vi "CMN_Algors.vi"(0 "ValueIn":string, 1 "file":path, 2 "algors":string[](array[string]), 3 "error in (no error)":errorcluster, 5 "action":T2(ring)) -> (7 "Value out":sgl format="%.6f", 9 "string value":string, 10 "error out":errorcluster)   [LabVIEW 2016]
uses:
  <vilib>/Utility/config.llb/Read Key (String).vi
  <vilib>/Utility/config.llb/NI_LVConfig.lvlib
panel:
  in  "algor":T1
  # "Hacer un <Window/SHOW DIAGRAM> para ver \nalgoritmos definidos o agregar uno nuevo"
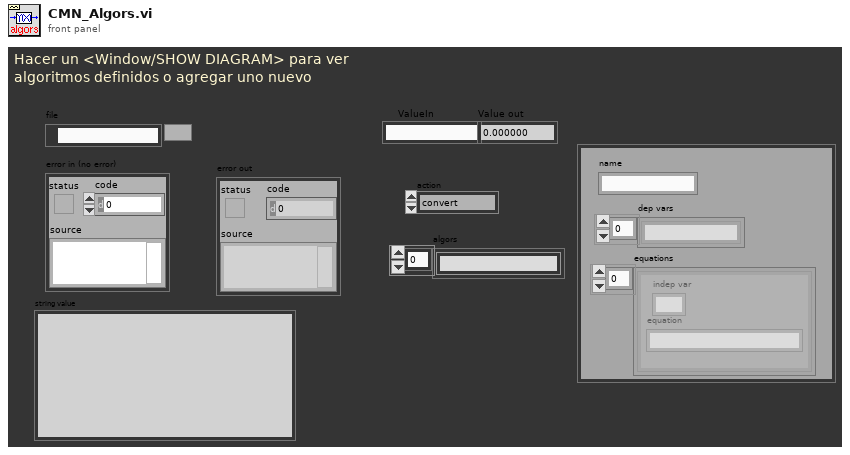
[diagram p1: front panel]
types:
  T1 = cluster{"name":string, "dep vars":string[], "equations":cluster{"indep var":string, "equation":string}[]}
  T2 = enum16{"convert", "read from file", "get", "clear all", "get all", "delete"}
  T3 = cluster{"name":string, "dep vars":string[], "equations":cluster{"indep var":string, "equation":string}[]}[]
  T4 = typedef "NI_LVConfig.lvlib/Config Data RefNum.ctl" = refnum<k1>
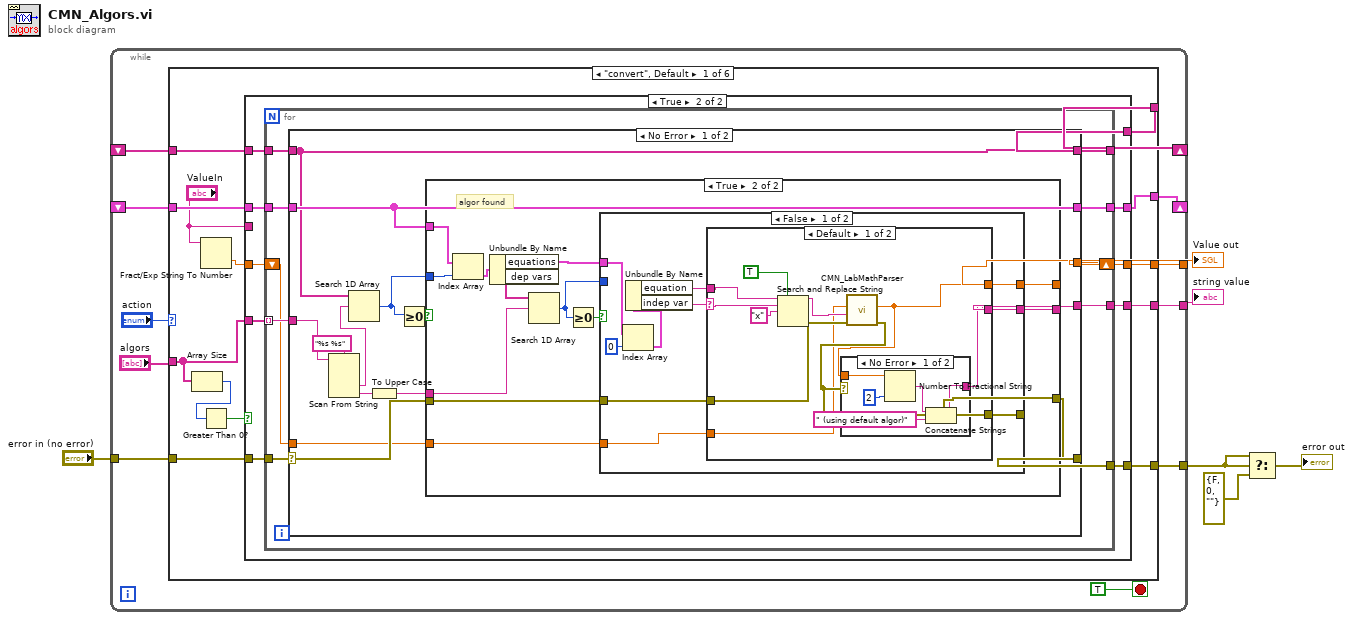
[diagram p0: block diagram]
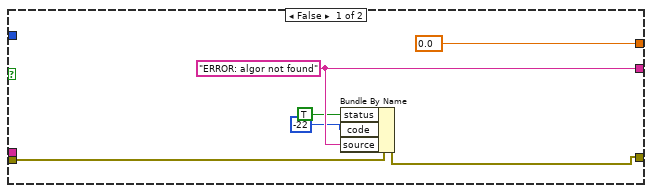
[diagram p3: hidden frame]
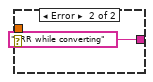
[diagram p4: hidden frame]
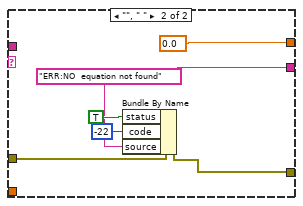
[diagram p5: hidden frame]
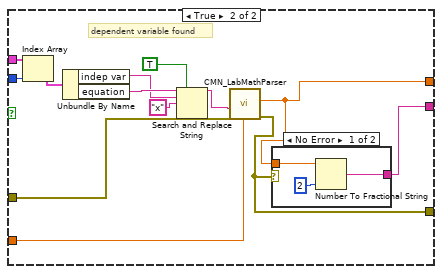
[diagram p6: hidden frame]
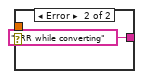
[diagram p7: hidden frame]
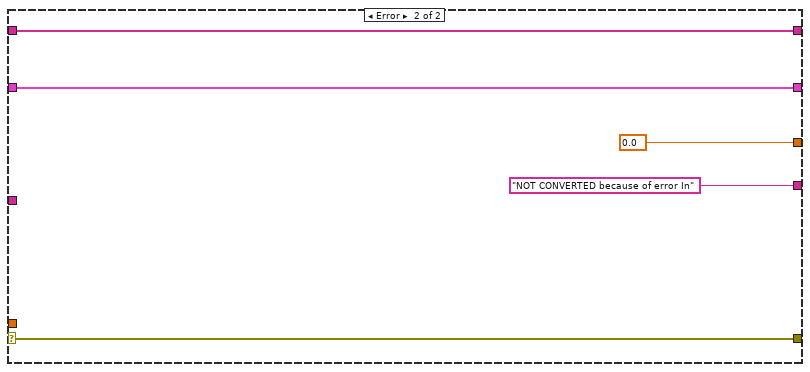
[diagram p8: hidden frame]
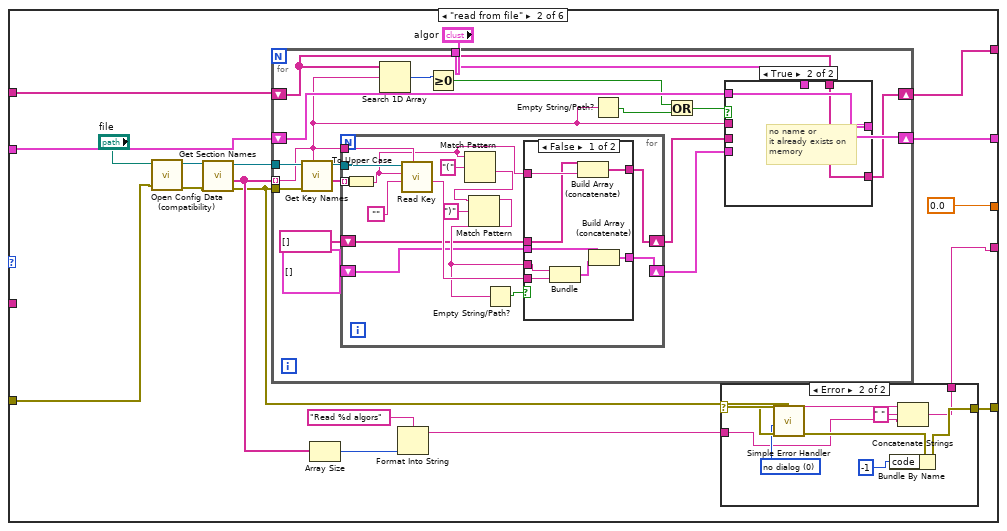
[diagram p9: hidden frame]
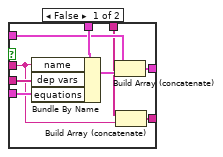
[diagram p11: hidden frame]
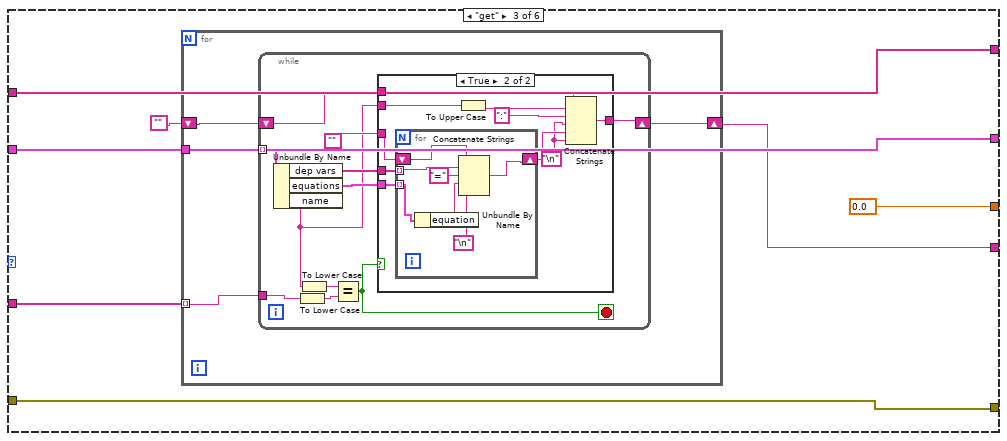
[diagram p13: hidden frame]
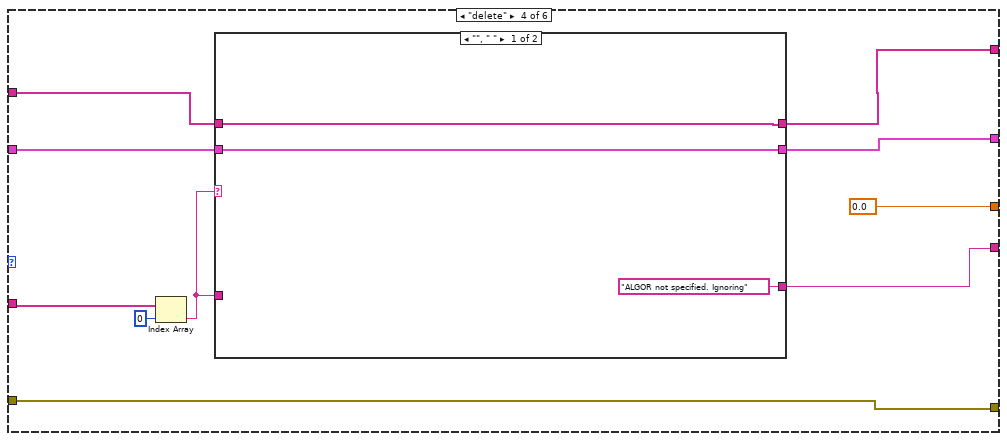
[diagram p15: hidden frame]
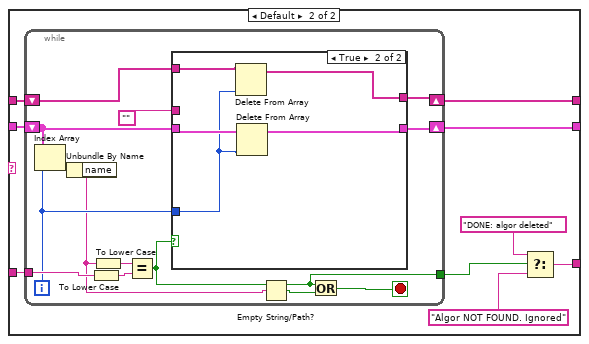
[diagram p16: hidden frame]
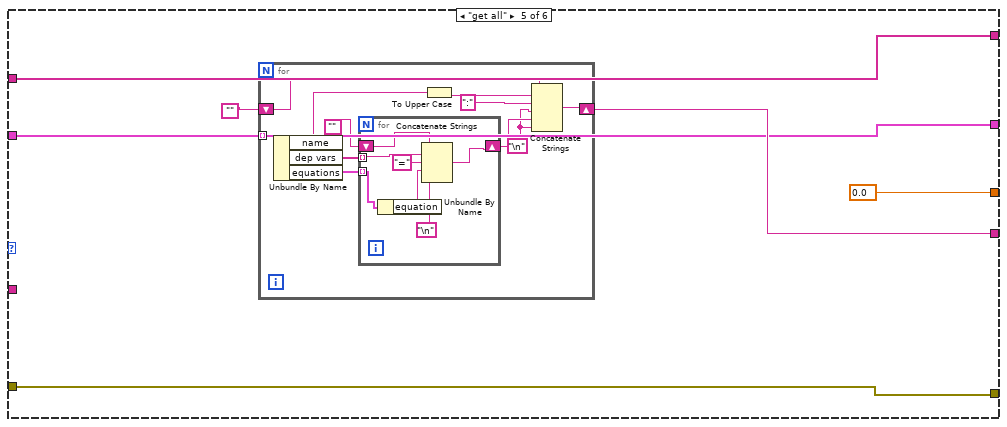
[diagram p18: hidden frame]
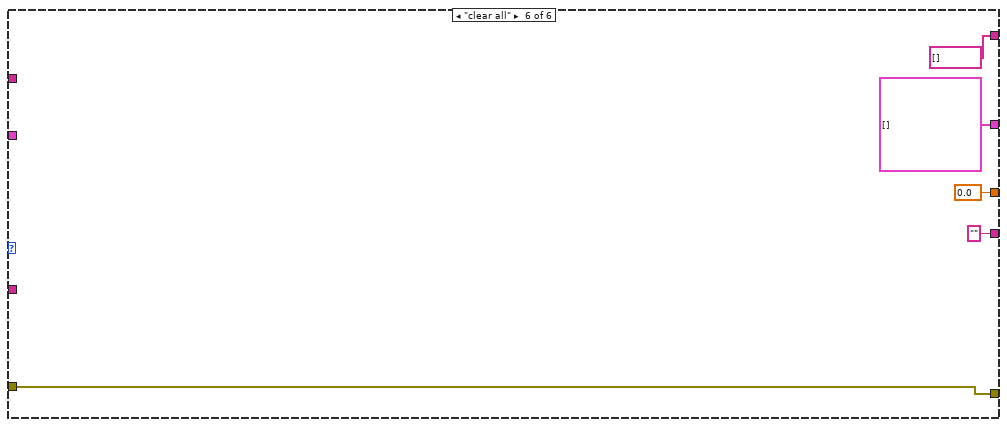
[diagram p19: hidden frame]
diagram:
  n1 = while {
    tunnel: "error in (no error)" -> [w17]
    tunnel: [w16] -> w3
    tunnel: [w15] -> w5
    tunnel: [w14] -> w4
    shift-right: [w8] -> _
    shift-left: _ -> [w11]
    shift-right: [w10] -> _
    shift-left: _ -> [w9]
    stop <- TRUE stop-if-true
    n2 = case shown="\"convert\", Default" "action" {
      tunnel: w17 -> [w30 w156 w230 w274 w310 w333]
      tunnel: [w29 w145 w230 w274 w310 w333] -> w16
      tunnel: [w23 0.0 ("y") 0.0 ("y") 0.0 ("y") 0.0 ("y") 0.0 ("y")] -> w15
      tunnel: [w28 w143 w227 w268 w313 "" ("source")] -> w14
      tunnel: w11 -> [w27 w153 w229 w271 w309 _]
      tunnel: [w25 w148 w231 w269 w311 string[] [] ("section names")] -> w10
      tunnel: w9 -> [w26 w149 w231 w270 w311 _]
      tunnel: [w24 w154 w229 w266 w309 T3 []] -> w8
      tunnel: "algors" -> [w22 _ w228 w273 _ _]
      frame "convert", Default {
        n3 = Array Size(array=w22) -> (size(s)=w21:i32)
        n4 = Fract/Exp String To Number(string="ValueIn") -> (number=w19:dbl)  [unwired: 4 out]
        n5 = Greater Than 0?(x=w21) -> (x > 0?=w20:bool)
        n6 = case shown="True" w20 {
          tunnel: w30 -> [w35 w45]
          tunnel: [w35 w44] -> w29
          tunnel: [w31 w43] -> w28
          tunnel: w27 -> [w33 w42]
          tunnel: w26 -> [w32 w41]
          tunnel: [w32 w40] -> w25
          tunnel: [w33 w39] -> w24
          tunnel: [w34 w38] -> w23
          tunnel: w19 -> [w34 w37]
          tunnel: w22 -> [_ w36]
          tunnel: "ValueIn" -> [w31 _]
          frame False {
            # "empty algor; just pass the value"
          }
          frame True {
            n7 = for {
              tunnel: w45 -> [w55]
              tunnel: [w54] -> w44
              tunnel: [w52] -> w43
              tunnel: w42 -> [w51]
              tunnel: w41 -> [w50]
              tunnel: [w49] -> w39
              tunnel: [w48] -> w40
              tunnel: w36 -> [w47] mode=indexing
              shift-right: [w53] -> w38
              shift-left: w37 -> [w46]
              n8 = case shown="No Error" w55 {
                selector: w55 -> [w65 w141]
                tunnel: [w67 0.0 ("y")] -> w53
                tunnel: [w64 w141] -> w54
                tunnel: [w66 "NOT CONVERTED because of error In"] -> w52
                tunnel: w51 -> [w63 w139]
                tunnel: w50 -> [w62 w138]
                tunnel: [w63 w139] -> w49
                tunnel: [w62 w138] -> w48
                tunnel: w47 -> [w57 _]
                tunnel: w46 -> [w56 _]
                frame No Error {
                  n9 = Scan From String(format string="%s %s", input string=w57) -> (output 1=w60:string, output 2=w59:string)  [unwired: 2 in, 5 out]
                  n10 = Search 1D Array(1D array=w62, element=w60) -> (index of element=w68:i32)  [unwired: 1 out]
                  n11 = To Upper Case(1:w59) -> (0:w58:string)
                  n12 = Greater Or Equal To 0?(x=w68) -> (x >= 0?=w69:bool)
                  n13 = case shown="True" w69 {
                    tunnel: w63 -> [_ w88]
                    tunnel: w68 -> [_ w87]
                    tunnel: [0.0 ("Result") w80] -> w67
                    tunnel: [w74 w79] -> w66
                    tunnel: w65 -> [w71 w78]
                    tunnel: [w70 w77] -> w64
                    tunnel: w58 -> [_ w84]
                    tunnel: w56 -> [_ w76]
                    frame False {
                      w74 = "ERROR: algor not found"
                      n14 = Bundle By Name(cluster=w71, "status"=TRUE, "code"=-22, "source"=w74) -> (w70:errorcluster)
                    }
                    frame True {
                      # "algor found"
                      n15 = Index Array(array=w88, index=w87) -> (element=w86:T1)
                      n16 = Unbundle By Name(w86) -> ("equations"=w82:cluster{"indep var":string, "equation":string}[], "dep vars"=w85:string[])
                      n17 = Search 1D Array(1D array=w85, element=w84) -> (index of element=w81:i32)  [unwired: 1 out]
                      n18 = Greater Or Equal To 0?(x=w81) -> (x >= 0?=w83:bool)
                      n19 = case shown="False" w83 {
                        tunnel: w82 -> [w94 w133]
                        tunnel: w81 -> [_ w132]
                        tunnel: [w96 w125] -> w80
                        tunnel: [w95 w124] -> w79
                        tunnel: w78 -> [w98 w123]
                        tunnel: [w97 w122] -> w77
                        tunnel: w76 -> [w89 w121]
                        frame False {
                          n20 = Index Array(array=w94, index=0) -> (element=w92:cluster{"indep var":string, "equation":string})
                          n21 = Unbundle By Name(w92) -> ("equation"=w90:string, "indep var"=w91:string)
                          n22 = case shown="Default" w91 {
                            selector: w91 -> [w105 _]
                            tunnel: w98 -> [w103 w120]
                            tunnel: [w102 w119] -> w97
                            tunnel: [w101 0.0 ("answer")] -> w96
                            tunnel: [w100 w115] -> w95
                            tunnel: w90 -> [w104 _]
                            tunnel: w89 -> [w99 _]
                            frame Default {
                              n23 = Search and Replace String(replace all?=TRUE ("replace all? (F)"), input string=w104, search string=w105, replace string="x" ("replace string (\"\")")) -> (result string=w107:string)  [unwired: 1 in, 6 out]
                              n24 = call "CMN_LabMathParser.vi"("error in (no error)"=w103, "expression"=w107, "x"=w99) -> ("error out"=w102:errorcluster, "answer"=w101:dbl)  [unwired: 7 out]
                              n25 = case shown="No Error" w102 {
                                tunnel: w101 -> [w112 _]
                                tunnel: [w109 "ERR while converting"] -> w100
                                frame No Error {
                                n26 = Number To Fractional String(number=w112, precision (6)=i16 2) -> (F-format string=w111:string)  [unwired: 2 out]
                                n27 = Concatenate Strings(w111, " (using default algor)" ("string")) -> (w109:string)
                                }
                                frame Error {
                                }
                              }
                            }
                            frame "", " " {
                              w115 = "ERR:NO  equation not found" ("source")
                              n28 = Bundle By Name(cluster=w120, "status"=TRUE, "code"=-22, "source"=w115) -> (w119:errorcluster)
                            }
                          }
                        }
                        frame True {
                          # "dependent variable found"
                          n29 = Index Array(array=w133, index=w132) -> (element=w128:cluster{"indep var":string, "equation":string})
                          n30 = Unbundle By Name(w128) -> ("indep var"=w126:string, "equation"=w127:string)
                          n31 = Search and Replace String(replace all?=TRUE ("replace all? (F)"), input string=w127, search string=w126, replace string="x" ("replace string (\"\")")) -> (result string=w130:string)  [unwired: 1 in, 6 out]
                          n32 = call "CMN_LabMathParser.vi"("error in (no error)"=w123, "expression"=w130, "x"=w121) -> ("error out"=w122:errorcluster, "answer"=w125:dbl)  [unwired: 7 out]
                          n33 = case shown="No Error" w122 {
                            tunnel: w125 -> [w135 _]
                            tunnel: [w134 "ERR while converting"] -> w124
                            frame No Error {
                              n34 = Number To Fractional String(number=w135, precision (6)=i16 2) -> (F-format string=w134:string)  [unwired: 2 out]
                            }
                            frame Error {
                            }
                          }
                        }
                      }
                    }
                  }
                }
                frame Error {
                }
              }
            }
          }
        }
      }
      frame "read from file" {
        n35 = call <vilib>:"Open Config Data (compatibility).vi"("error in (no error)"=w156, "configuration file path"="file") -> ("error out"=w160:errorcluster, "refnum"=w159:T4)  [unwired: 7 in, 1 out]
        n36 = call <vilib>:"Get Section Names.vi"("error in (no error)"=w160, "refnum"=w159) -> ("error out"=w146:errorcluster, "section names"=w150:string[], "refnum out"=w158:T4)  [unwired: 7 out]
        n37 = for {
          tunnel: w146 -> [w187]
          tunnel: w158 -> [w188]
          tunnel: w150 -> [w178] mode=indexing
          tunnel: "algor" -> [w189]
          shift-right: [w184] -> w154
          shift-left: w153 -> [w183]
          shift-right: [w172] -> w148
          shift-left: w149 -> [w173]
          n38 = call <vilib>:"Get Key Names.vi"("section"=w178, "error in (no error)"=w187, "refnum"=w188) -> ("key names"=w186:string[], "refnum out"=w185:T4)  [unwired: 7 out]
          n39 = for {
            tunnel: w186 -> [w205] mode=indexing
            tunnel: w185 -> [w215]
            tunnel: w178 -> [w213]
            shift-right: [w207] -> w181
            shift-left: cluster{"String":string, "value":string}[] [] -> [w206]
            shift-right: [w204] -> w180
            shift-left: string[] [] -> [w203]
            n40 = To Upper Case(1:w205) -> (0:w201:string)
            n41 = call-poly <vilib>:"Read Key.vi"("section"=w213, "default value"="", "key"=w201, "refnum"=w215) -> ("value"=w209:string)  [unwired: 2 in, 5 out]
            n42 = Match Pattern(string=w201, regular expression="(") -> (after substring=w211:string)  [unwired: 4 out]
            n43 = Match Pattern(string=w211, regular expression=")") -> (before substring=w208:string)  [unwired: 4 out]
            n44 = Empty String/Path?(string/path=w208) -> (empty?=w202:bool)
            n45 = case shown="False" w202 {
              tunnel: w209 -> [w223 _]
              tunnel: w208 -> [w222 _]
              tunnel: [w220 w225] -> w207
              tunnel: w206 -> [w219 w225]
              tunnel: w201 -> [w218 _]
              tunnel: [w217 w224] -> w204
              tunnel: w203 -> [w216 w224]
              frame False {
                n46 = Bundle(w222, "value"=w223) -> (w221:cluster{string, "value":string})  [unwired: 1 out]
                n47 = Build Array (concatenate)(w216, w218) -> (w217:string[])
                n48 = Build Array (concatenate)(w219, w221) -> (w220:cluster{"String":string, "value":string}[])
              }
              frame True {
              }
            }
          }
          n49 = Search 1D Array(1D array=w173, element=w178) -> (index of element=w177:i32)  [unwired: 1 out]
          n50 = Greater Or Equal To 0?(x=w177) -> (x >= 0?=w174:bool)
          n51 = Empty String/Path?(string/path=w178) -> (empty?=w175:bool)
          n52 = Or(x=w174, y=w175) -> (x .or. y?=w176:bool)
          n53 = case shown="True" w176 {
            tunnel: w189 -> [w198 _]
            tunnel: w178 -> [w191 _]
            tunnel: w181 -> [w197 _]
            tunnel: w180 -> [w196 _]
            tunnel: [w194 w200] -> w184
            tunnel: w183 -> [w193 w200]
            tunnel: w173 -> [w192 w199]
            tunnel: [w190 w199] -> w172
            frame False {
              n54 = Bundle By Name(cluster=w198, "name"=w191, "dep vars"=w196, "equations"=w197) -> (w195:T1)
              n55 = Build Array (concatenate)(w193, w195) -> (w194:T3)
              n56 = Build Array (concatenate)(w192, w191) -> (w190:string[])
            }
            frame True {
              # "no name or\nit already exists on\nmemory"
            }
          }
        }
        n57 = Array Size(array=w150) -> (size(s)=w152:i32)
        n58 = Format Into String(format string="Read %d algors", w152) -> (resulting string=w144:string)  [unwired: 2 in, 1 out]
        n59 = case shown="Error" w146 {
          selector: w146 -> [w162 w171]
          tunnel: [w162 w168] -> w145
          tunnel: w144 -> [w161 w164]
          tunnel: [w161 w163] -> w143
          frame No Error {
          }
          frame Error {
            w170 = u16 0 items=["no dialog", "OK message", "continue or stop message"] ("type of dialog (OK msg:1)")
            n60 = call <vilib>:"Simple Error Handler.vi"("type of dialog (OK msg:1)"=w170, "error in (no error)"=w171) -> ("error out"=w169:errorcluster, "message"=w166:string)  [unwired: 6 out]
            n61 = Bundle By Name(cluster=w169, "code"=-1) -> (w168:errorcluster)
            n62 = Concatenate Strings(w166, " " ("string"), w164) -> (w163:string)
          }
        }
      }
      frame "get" {
        n63 = for {
          tunnel: w229 -> [w236]
          tunnel: w228 -> [w235] mode=indexing
          shift-right: [w234] -> w227
          shift-left: "" -> [w233]
          n64 = while {
            tunnel: w236 -> [w247] mode=indexing
            shift-right: [w243] -> w234
            shift-left: w233 -> [w242]
            tunnel: w235 -> [w241]
            stop <- w238 stop-if-true
            n65 = Unbundle By Name(w247) -> ("dep vars"=w246:string[], "equations"=w245:cluster{"indep var":string, "equation":string}[], "name"=w237:string)
            n66 = To Lower Case(string=w241) -> (all lower case string=w239:string)
            n67 = To Lower Case(string=w237) -> (all lower case string=w240:string)
            n68 = Equal?(x=w240, y=w239) -> (x = y?=w238:bool)
            n69 = case shown="True" w238 {
              tunnel: w246 -> [_ w258]
              tunnel: w245 -> [_ w257]
              tunnel: "" -> [_ w256]
              tunnel: w237 -> [_ w255]
              tunnel: [w248 w252] -> w243
              tunnel: w242 -> [w248 w251]
              frame False {
              }
              frame True {
                w249 = "\n"
                n70 = for {
                  tunnel: w258 -> [w265] mode=indexing
                  tunnel: w257 -> [w263] mode=indexing
                  shift-right: [w260] -> w250
                  shift-left: w256 -> [w259]
                  n71 = Unbundle By Name(w263) -> ("equation"=w262:string)
                  n72 = Concatenate Strings(w259, w265, "=" ("string"), w262, "\n") -> (w260:string)
                }
                n73 = To Upper Case(1:w255) -> (0:w254:string)
                n74 = Concatenate Strings(w251, w254, ":" ("string"), w249, w250, w249) -> (w252:string)
              }
            }
          }
        }
      }
      frame "delete" {
        n75 = Index Array(array=w273, index=0) -> (element=w267:string)
        n76 = case shown="\"\", \" \"" w267 {
          tunnel: w267 -> [_ w287]
          tunnel: w271 -> [w277 w286]
          tunnel: w270 -> [w278 w285]
          tunnel: [w278 w284] -> w269
          tunnel: ["ALGOR not specified. Ignoring" ("f") w280] -> w268
          tunnel: [w277 w279] -> w266
          frame "", " " {
          }
          frame Default {
            n77 = while {
              shift-right: [w300] -> w284
              shift-left: w285 -> [w299]
              tunnel: w287 -> [w298]
              shift-right: [w293] -> w279
              shift-left: w286 -> [w294]
              tunnel: [w288] -> w283
              i -> [w292]
              stop <- w291 stop-if-true
              n78 = Index Array(array=w294, index=w292) -> (element=w295:T1)
              n79 = Unbundle By Name(w295) -> ("name"=w290:string)
              n80 = To Lower Case(string=w298) -> (all lower case string=w296:string)
              n81 = To Lower Case(string=w290) -> (all lower case string=w297:string)
              n82 = Equal?(x=w297, y=w296) -> (x = y?=w288:bool)
              n83 = case shown="True" w288 {
                tunnel: "" -> [_ _]
                tunnel: [w303 w305] -> w300
                tunnel: w299 -> [w303 w308]
                tunnel: w294 -> [w302 w307]
                tunnel: [w302 w304] -> w293
                tunnel: w292 -> [_ w306]
                frame False {
                }
                frame True {
                  n84 = Delete From Array(array=w308, index=w306) -> (array with subset deleted=w305:string[])  [unwired: 1 in, 1 out]
                  n85 = Delete From Array(array=w307, index=w306) -> (array with subset deleted=w304:T3)  [unwired: 1 in, 1 out]
                }
              }
              n86 = Empty String/Path?(string/path=w290) -> (empty?=w289:bool)
              n87 = Or(x=w288, y=w289) -> (x .or. y?=w291:bool)
            }
            n88 = Select(t="DONE: algor deleted", s=w283, f="Algor NOT FOUND. Ignored") -> (s? t:f=w280:string)
          }
        }
      }
      frame "get all" {
        n89 = for {
          tunnel: w309 -> [w325] mode=indexing
          shift-right: [w318] -> w313
          shift-left: "" -> [w317]
          w315 = "\n"
          n90 = Unbundle By Name(w325) -> ("name"=w321:string, "dep vars"=w324:string[], "equations"=w323:cluster{"indep var":string, "equation":string}[])
          n91 = for {
            tunnel: w324 -> [w332] mode=indexing
            tunnel: w323 -> [w330] mode=indexing
            shift-right: [w327] -> w316
            shift-left: "" -> [w326]
            n92 = Unbundle By Name(w330) -> ("equation"=w329:string)
            n93 = Concatenate Strings(w326, w332, "=" ("string"), w329, "\n") -> (w327:string)
          }
          n94 = To Upper Case(1:w321) -> (0:w320:string)
          n95 = Concatenate Strings(w317, w320, ":" ("string"), w315, w316, w315) -> (w318:string)
        }
      }
      frame "clear all" {
      }
    }
  }
  "Value out" <- w5
  "string value" <- w4
  n96 = Select(t=w3, s=w3, f=errorcluster {"status"=FALSE, "code"=0, "source"=""}) -> (s? t:f=→"error out":errorcluster)
